vi "Current_Training_UI.vi"() -> ()   [LabVIEW 2021]
uses:
  SerialVIs/Processors.ctl
panel:
  out "Motor Value":i32
  in  "Quit":bool
  out "Training String":string
  out "Tab Control":enum32{"Welcome", "View", "Train"}(tab)
  in  "Ready":bool
  out "new picture":picture
  out "Motor Position View":dbl(knob) scale=0.0..180.0 scale format="%^#_3g"
  in  "TRAIN":bool
  out "Light Intensity % View":dbl(slide) scale=0.0..100.0
  out "?":u32(colorbox)
  out "new picture 4":picture
  in  "Done":bool
  in  "Motor Position":dbl(knob) scale=0.0..180.0 scale format="%^#_3g"
  out "Light Intensity %":dbl(slide) scale=0.0..100.0
  in  "Training Data":bool
  in  "Upload":bool
  out "Light Intensity 2":u32(colorbox)
  out "new picture 2":picture
  out "new picture 3":picture
  in  "Done 2":bool
  out "Upload String":string
  out "concatenated string":string
  out "read buffer":string
  out "Motor":string
  out "Sensor":string
  out "Type":string
  out "Name":string
  out "read terminal buffer - view":string
  out "Serial Settings:Number of Bytes at Serial Port 2":u32
  out "read buffer 2":string
  # "help button pops up a help message"
  # "1"
  # "2"
  # "5"
  # "3"
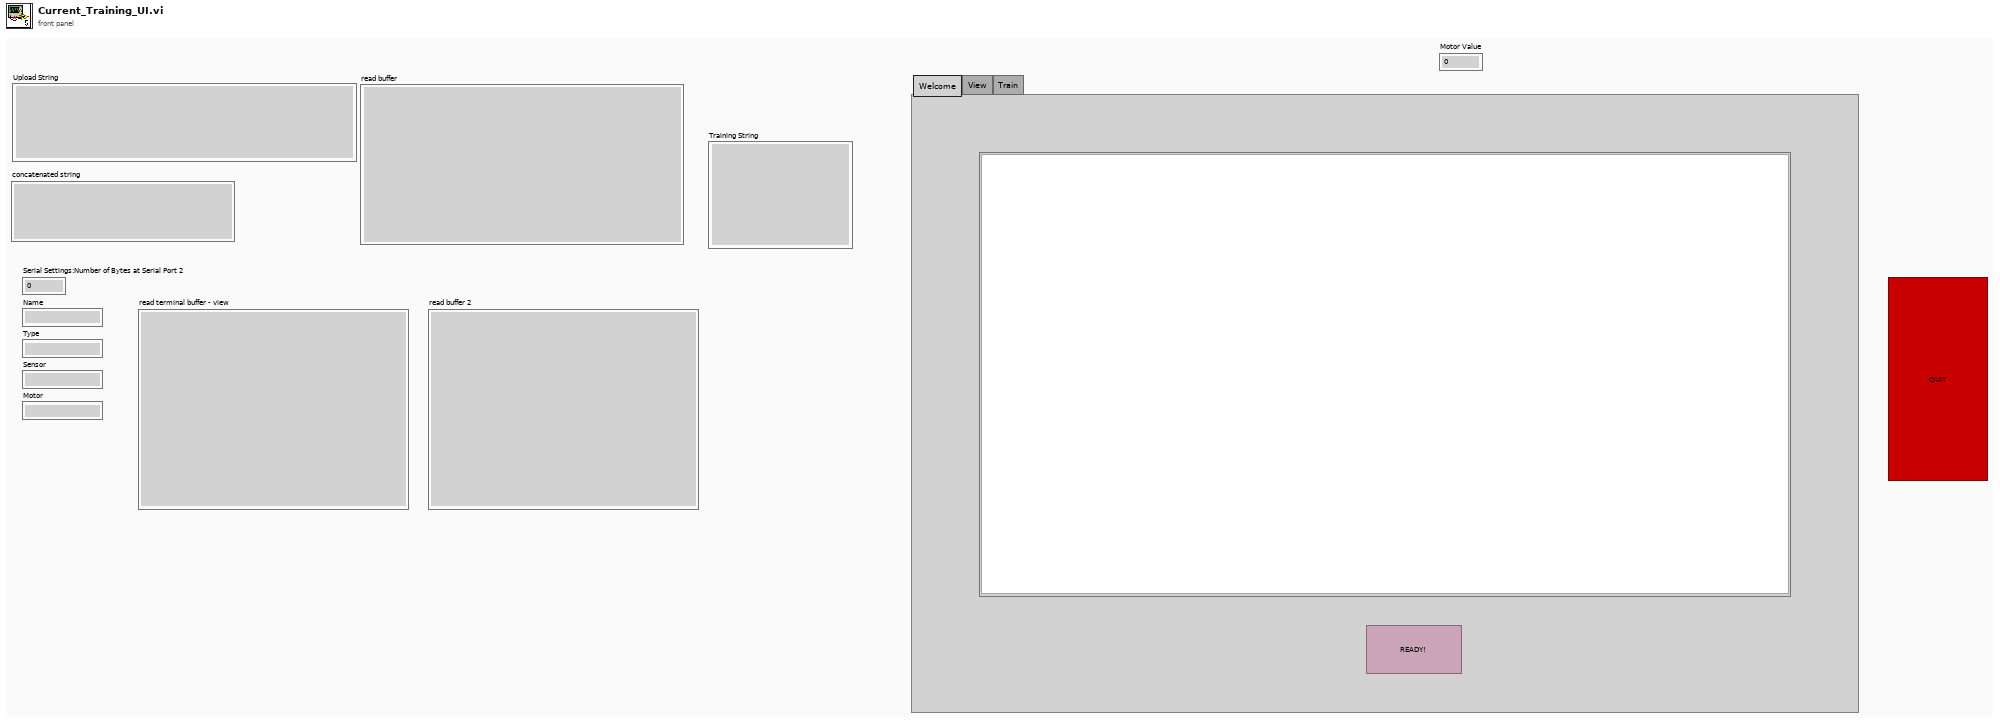
[diagram p1: front panel]
types:
  T1 = typedef "Processors.ctl" = enum16{"SPIKE", "Pi", "Pi_ssh", "OpenMV"}
  T2 = typedef "PythonCtrl.ctl" = cluster{"session":refnum<k35>, "PyPath":path, "Processor":enum16{"SPIKE", "Pi", "Pi_ssh"}}
  T3 = typedef "imagedata.ctl" = cluster{"image type":i32, "image depth":i32, "image":u8[], "mask":u8[], "colors":u32[], "Rectangle":cluster{"left":i16, "top":i16, "right":i16, "bottom":i16}}
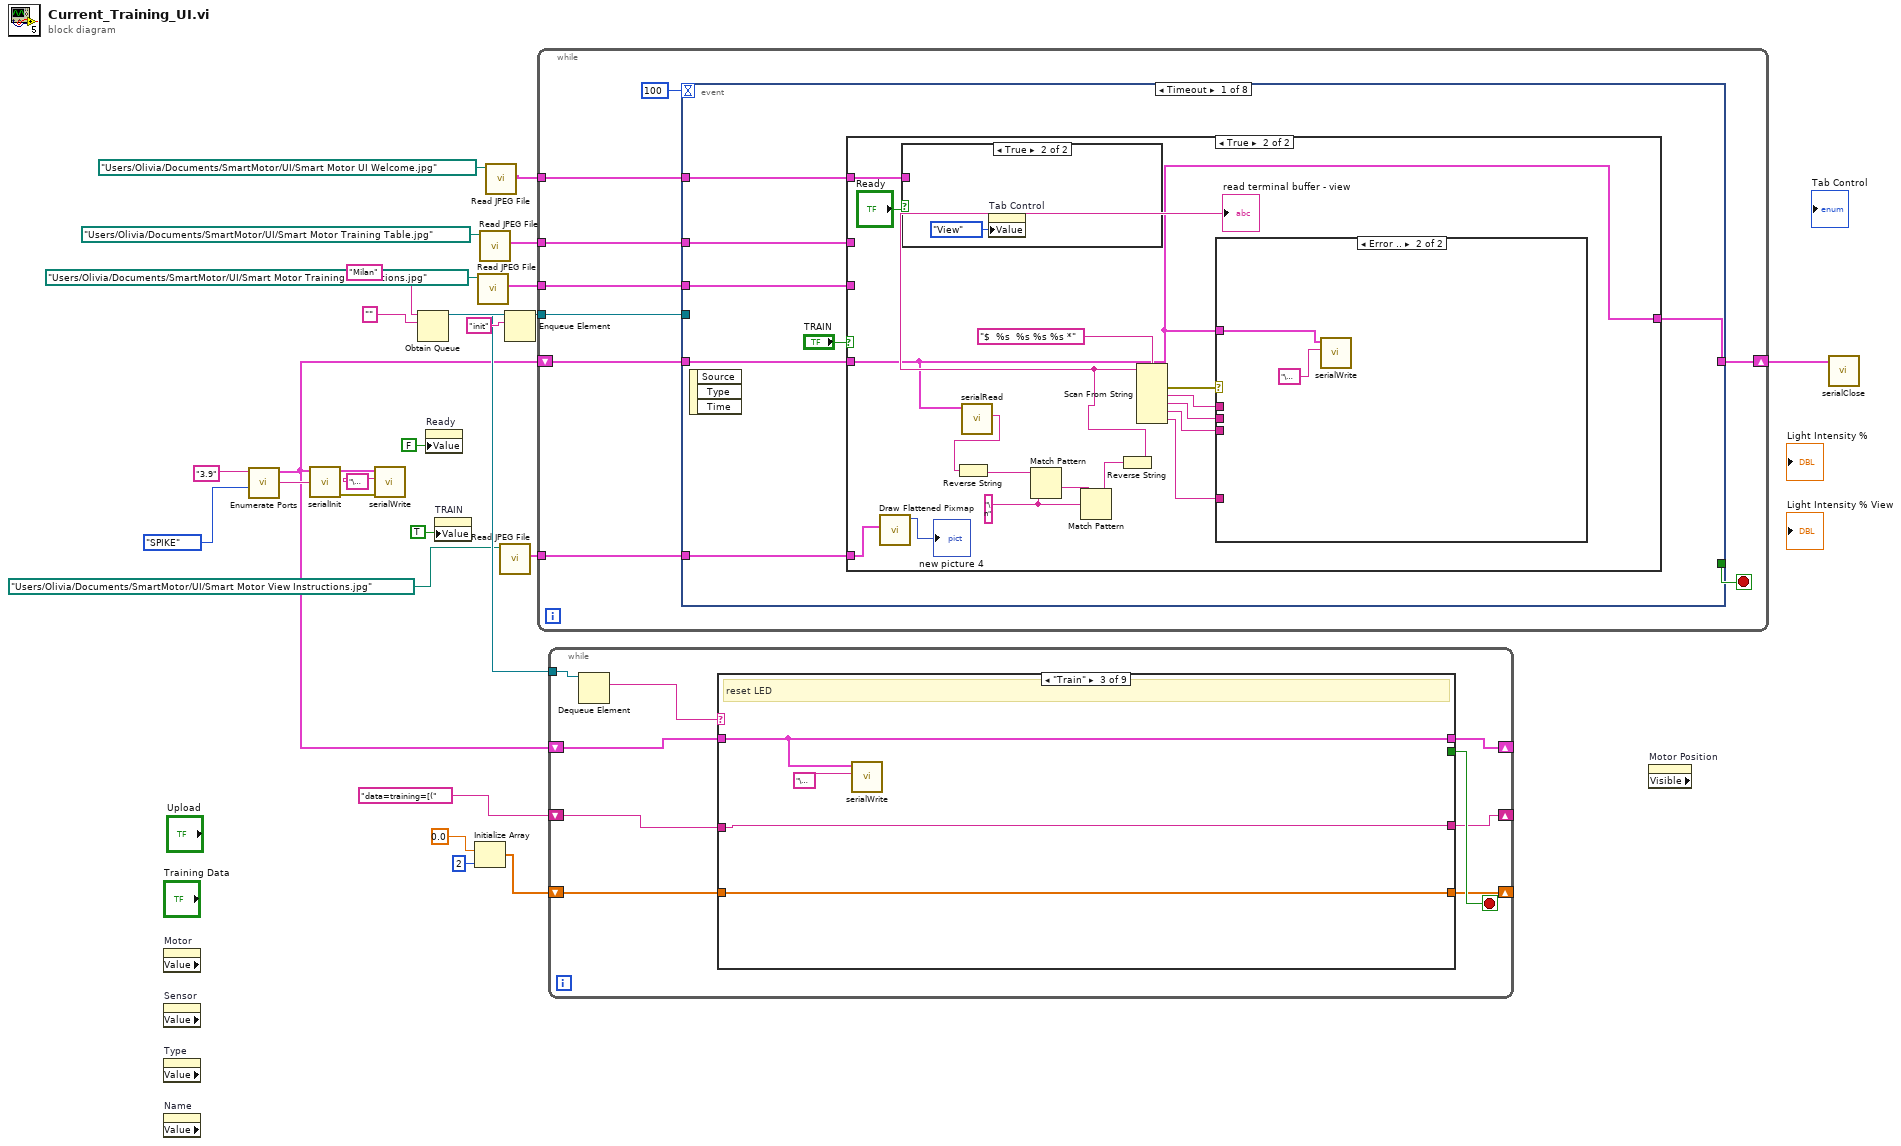
[diagram p0: block diagram]
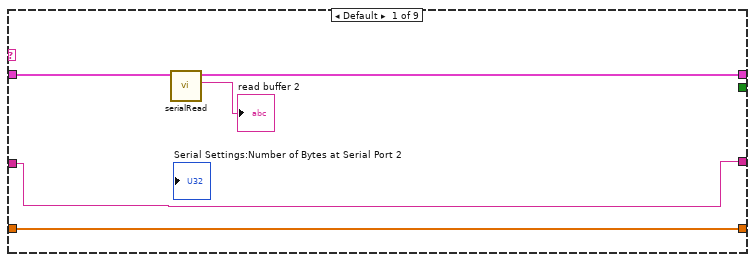
[diagram p2: hidden frame]
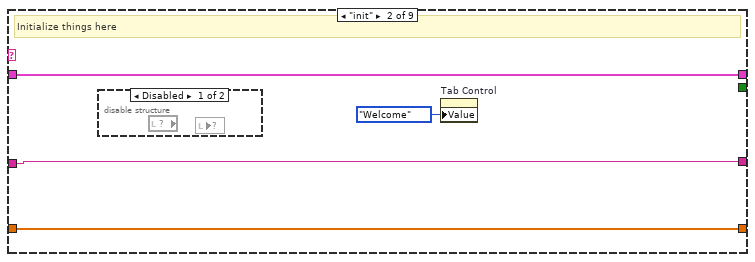
[diagram p3: hidden frame]
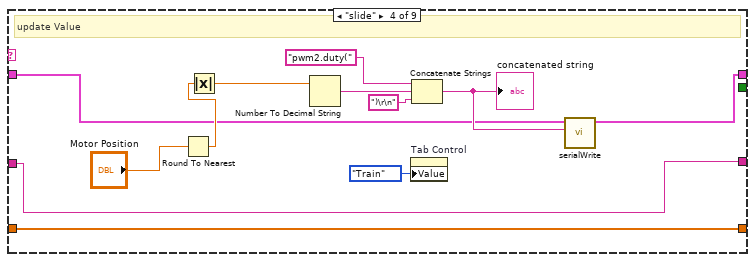
[diagram p5: hidden frame]
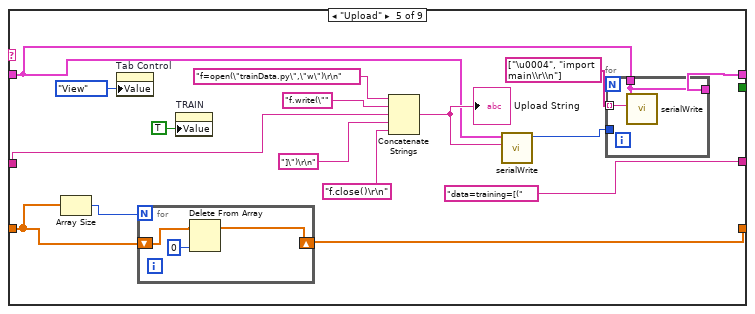
[diagram p6: hidden frame]
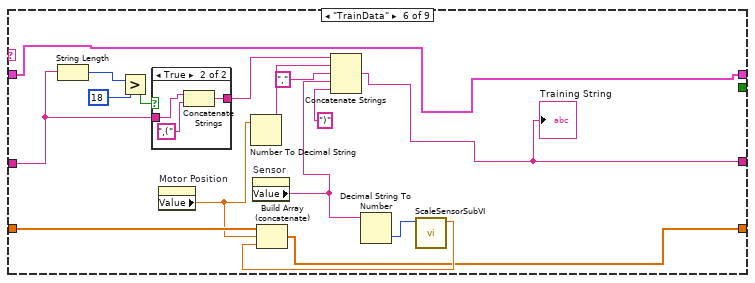
[diagram p7: hidden frame]
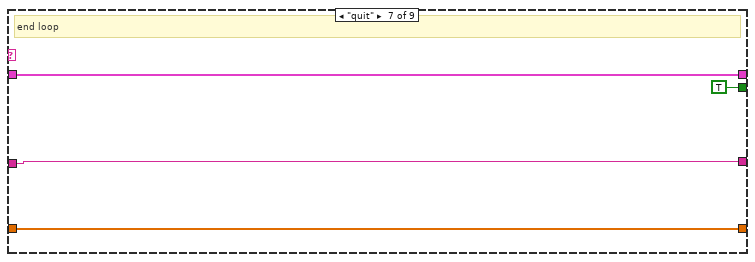
[diagram p9: hidden frame]
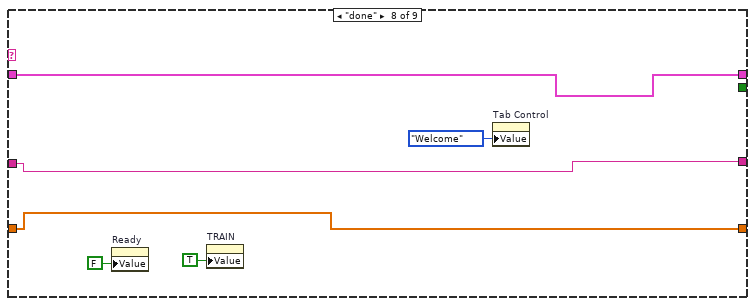
[diagram p10: hidden frame]
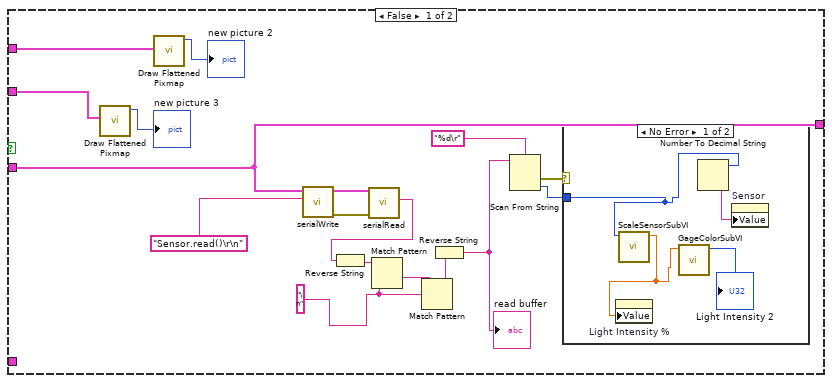
[diagram p12: hidden frame]
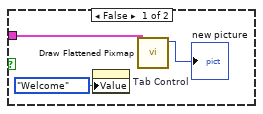
[diagram p14: hidden frame]
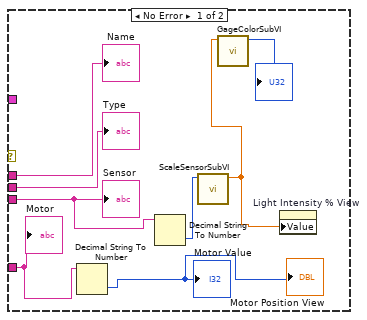
[diagram p15: hidden frame]
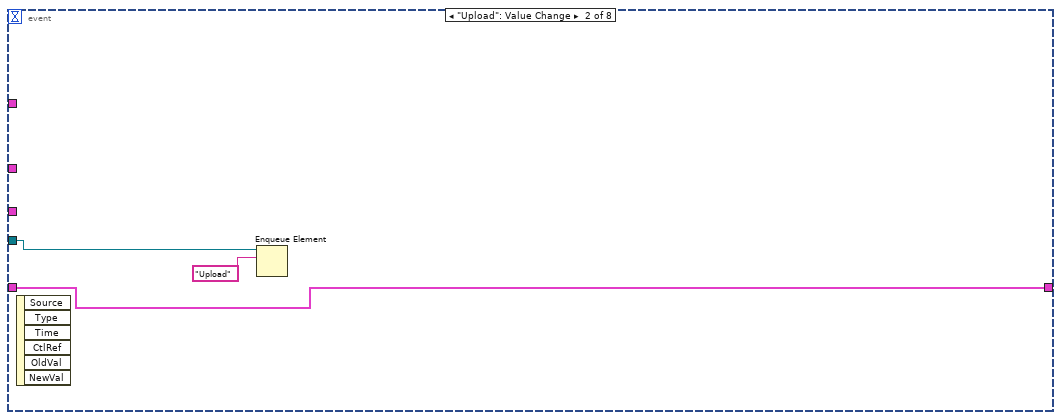
[diagram p16: hidden frame]
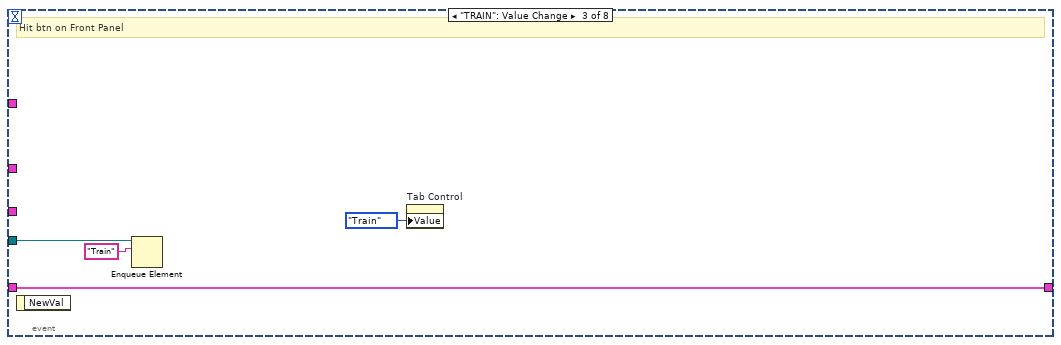
[diagram p17: hidden frame]
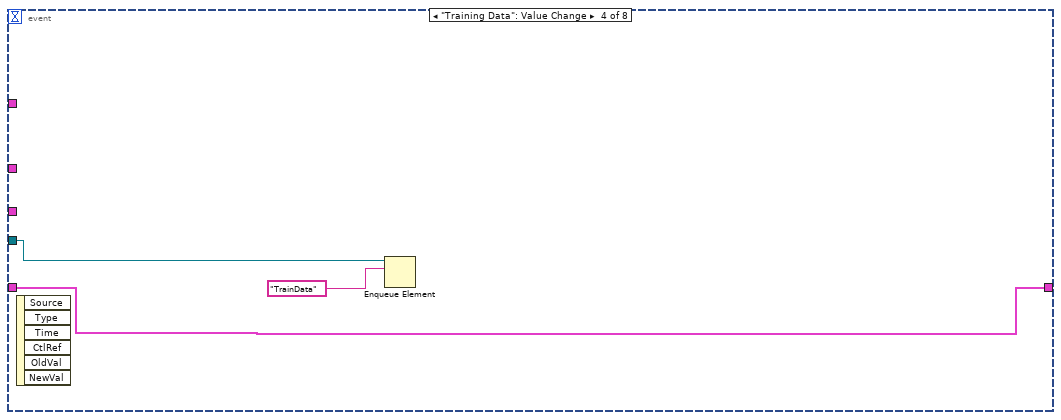
[diagram p18: hidden frame]
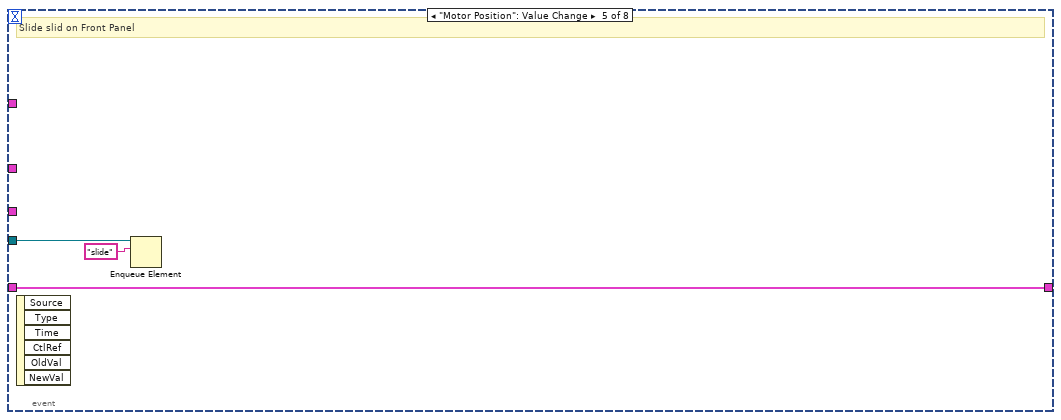
[diagram p19: hidden frame]
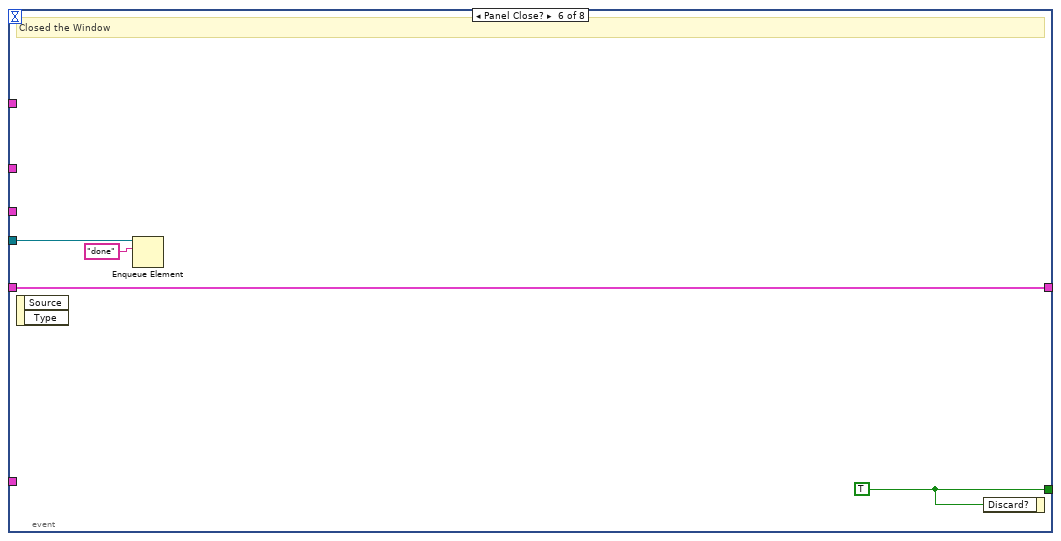
[diagram p20: hidden frame]
diagram:
  n1 = property on="Motor" class="Str" props=["Value"]() -> ()  [unwired: 2 in, 3 out]
  n2 = property on="Sensor" class="Str" props=["Value"]() -> ()  [unwired: 2 in, 3 out]
  n3 = property on="Type" class="Str" props=["Value"]() -> ()  [unwired: 2 in, 3 out]
  n4 = property on="Name" class="Str" props=["Value"]() -> ()  [unwired: 2 in, 3 out]
  n5 = call "Enumerate Ports.vi"("Processor"=Processors."SPIKE", "Python version"="3.9") -> ("guess"=w17:string, "Python"=w14:T2)  [unwired: 5 in, 3 out]
  n6 = call "serialInit.vi"("Port"=w17, "Python"=w14) -> ("error out"=w16:errorcluster)  [unwired: 8 in, 1 out]
  n7 = call "serialWrite.vi"("error in (no error)"=w16, "text"="\u0004" ("write buffer"), "Python"=w14) -> ()  [unwired: 7 in, 2 out]
  n8 = Obtain Queue(name (unnamed)="Milan", element data type="") -> (queue out=w26:refnum<queue>)  [unwired: 3 in, 2 out]
  n9 = property on="Ready" class="Bool (strict)"("Value"=FALSE ("Ready")) -> ()  [unwired: 2 in, 2 out]
  n10 = property on="TRAIN" class="Bool (strict)"("Value"=TRUE ("Train")) -> ()  [unwired: 2 in, 2 out]
  n11 = Initialize Array(0.0 ("element"), 2 ("dimension size")) -> (w2:dbl[])
  n12 = call <vilib>:"Read JPEG File.vi"("path to JPEG file"=path "/Users/Olivia/Documents/SmartMotor/UI/Smart Motor Training Instructions.jpg") -> ("image data"=w9:T3)  [unwired: 8 in, 2 out]
  n13 = call <vilib>:"Read JPEG File.vi"("path to JPEG file"=path "/Users/Olivia/Documents/SmartMotor/UI/Smart Motor Training Table.jpg") -> ("image data"=w11:T3)  [unwired: 8 in, 2 out]
  n14 = call <vilib>:"Read JPEG File.vi"("path to JPEG file"=path "/Users/Olivia/Documents/SmartMotor/UI/Smart Motor UI Welcome.jpg") -> ("image data"=w5:T3)  [unwired: 8 in, 2 out]
  n15 = call <vilib>:"Read JPEG File.vi"("path to JPEG file"=path "/Users/Olivia/Documents/SmartMotor/UI/Smart Motor View Instructions.jpg") -> ("image data"=w7:T3)  [unwired: 8 in, 2 out]
  n16 = Enqueue Element(queue=w26, element="init") -> (queue out=w22:refnum<queue>)  [unwired: 2 in, 2 out]
  n17 = while {
    tunnel: w22 -> [w35]
    shift-right: [w32] -> w13
    shift-left: w14 -> [w33]
    tunnel: w5 -> [w30]
    tunnel: w11 -> [w29]
    tunnel: w9 -> [w28]
    tunnel: w7 -> [w27]
    stop <- w34 stop-if-true
    n18 = event shown="[0] Timeout" {
      selector: _ -> [_ _ _ _ _ _ _ _]
      dyn-events: _ -> [_ _ _ _ _ _ _ _]
      timeout: 100 -> [_ _ _ _ _ _ _ _]
      tunnel: w35 -> [_ w96 w99 w102 w105 w109 w113 w116]
      tunnel: [_ _ _ _ _ w108 TRUE ("Discard?") _] -> w34
      tunnel: w33 -> [w40 w94 w98 w101 w104 w107 w111 w115]
      tunnel: [w41 w94 w98 w101 w104 w107 w111 w115] -> w32
      tunnel: w30 -> [w39 _ _ _ _ _ _ _]
      tunnel: w29 -> [w38 _ _ _ _ _ _ _]
      tunnel: w28 -> [w37 _ _ _ _ _ _ _]
      tunnel: w27 -> [w36 _ _ _ _ _ _ _]
      event Timeout {
        n19 = event-data() -> ()  [unwired: 1 in, 3 out]
        n20 = case shown="True" "TRAIN" {
          tunnel: w40 -> [w53 w63]
          tunnel: [w53 w63] -> w41
          tunnel: w39 -> [_ w66]
          tunnel: w38 -> [w45 _]
          tunnel: w37 -> [w43 _]
          tunnel: w36 -> [_ w64]
          frame False {
            w50 = "\n" ("regular expression")
            n21 = call <vilib>:"Draw Flattened Pixmap.vi"("image data"=w43) -> ("new picture"=→"new picture 3":picture)  [unwired: 8 in]
            n22 = call <vilib>:"Draw Flattened Pixmap.vi"("image data"=w45) -> ("new picture"=→"new picture 2":picture)  [unwired: 8 in]
            n23 = call "serialWrite.vi"("text"="Sensor.read()\r\n" ("write buffer"), "Python"=w53) -> ("error out"=w54:errorcluster)  [unwired: 8 in, 1 out]
            n24 = call "serialRead.vi"("error in (no error)"=w54, "Python"=w53) -> ("Reply"=w47:string)  [unwired: 7 in, 2 out]
            n25 = Reverse String(1:w47) -> (0:w52:string)
            n26 = Match Pattern(string=w52, regular expression=w50) -> (after substring=w51:string)  [unwired: 1 in, 3 out]
            n27 = Match Pattern(string=w51, regular expression=w50) -> (before substring=w49:string)  [unwired: 1 in, 3 out]
            n28 = Reverse String(1:w49) -> (0:w48:string)
            "read buffer" <- w48
            n29 = Scan From String(format string="%d\r", input string=w48) -> (error out=w58:errorcluster, output 1=w57:i32)  [unwired: 3 in, 2 out]
            n30 = case shown="No Error" w58 {
              tunnel: w57 -> [w60 _]
              frame No Error {
                n31 = call "ScaleSensorSubVI.vi"("Numeric in"=w60) -> ("Numeric out"=w59:dbl)  [unwired: 10 in]
                n32 = property on="Light Intensity %" class="Slide (strict)"("Value"=w59) -> ()  [unwired: 2 in, 2 out]
                n33 = call "GageColorSubVI.vi"("Numeric"=w59) -> ("Color Box"=→"Light Intensity 2":u32)  [unwired: 10 in]
                n34 = Number To Decimal String(number=w60) -> (decimal integer string=w62:string)  [unwired: 1 in]
                n35 = property on="Sensor" class="Str"("Value"=w62) -> ()  [unwired: 2 in, 2 out]
              }
              frame Error {
              }
            }
          }
          frame True {
            w70 = "\n" ("regular expression")
            n36 = call <vilib>:"Draw Flattened Pixmap.vi"("image data"=w64) -> ("new picture"=→"new picture 4":picture)  [unwired: 8 in]
            n37 = case shown="True" "Ready" {
              tunnel: w66 -> [w81 _]
              frame False {
                n38 = property on="Tab Control" class="TabCtl (strict)"("Value"=enum32{"Welcome", "View", "Train"}."Welcome" ("Tab Control")) -> ()  [unwired: 2 in, 2 out]
                n39 = call <vilib>:"Draw Flattened Pixmap.vi"("image data"=w81) -> ("new picture"=→"new picture":picture)  [unwired: 8 in]
              }
              frame True {
                n40 = property on="Tab Control" class="TabCtl (strict)"("Value"=enum32{"Welcome", "View", "Train"}."View" ("Tab Control")) -> ()  [unwired: 2 in, 2 out]
              }
            }
            n41 = call "serialRead.vi"("Python"=w63) -> ("Reply"=w73:string)  [unwired: 8 in, 2 out]
            n42 = Reverse String(1:w73) -> (0:w72:string)
            n43 = Match Pattern(string=w72, regular expression=w70) -> (after substring=w71:string)  [unwired: 1 in, 3 out]
            n44 = Match Pattern(string=w71, regular expression=w70) -> (before substring=w69:string)  [unwired: 1 in, 3 out]
            n45 = Reverse String(1:w69) -> (0:w68:string)
            "read terminal buffer - view" <- w68
            n46 = Scan From String(format string="$  %s  %s %s %s *", input string=w68) -> (error out=w79:errorcluster, output 1=w75:string, output 2=w76:string, output 3=w77:string, output 4=w78:string)  [unwired: 6 in, 2 out]
            n47 = case shown="Error .." w79 {
              tunnel: w75 -> [w91 _]
              tunnel: w76 -> [w90 _]
              tunnel: w77 -> [w89 _]
              tunnel: w78 -> [w85 _]
              tunnel: w63 -> [_ w93]
              frame No Error {
                n48 = Decimal String To Number(string=w85) -> (number=→"Motor Value" →"Motor Position View":i32)  [unwired: 2 in, 1 out]
                n49 = Decimal String To Number(string=w89) -> (number=w88:i32)  [unwired: 2 in, 1 out]
                n50 = call "ScaleSensorSubVI.vi"("Numeric in"=w88) -> ("Numeric out"=w86:dbl)  [unwired: 10 in]
                n51 = call "GageColorSubVI.vi"("Numeric"=w86) -> ("Color Box"=→"?":u32)  [unwired: 10 in]
                n52 = property on="Light Intensity % View" class="Slide (strict)"("Value"=w86) -> ()  [unwired: 2 in, 2 out]
                "Name" <- w91
                "Type" <- w90
                "Sensor" <- w89
                "Motor" <- w85
              }
              frame Error {
                n53 = call "serialWrite.vi"("text"="\u0003", "Python"=w93) -> ()  [unwired: 8 in, 2 out]
              }
            }
          }
        }
      }
      event "Upload": Value Change {
        n54 = event-data() -> ()  [unwired: 1 in, 6 out]
        n55 = Enqueue Element(queue=w96, element="Upload") -> ()  [unwired: 2 in, 3 out]
      }
      event "TRAIN": Value Change {
        # "Hit btn on Front Panel"
        n56 = event-data() -> ()  [unwired: 1 in, 1 out]
        n57 = Enqueue Element(queue=w99, element="Train") -> ()  [unwired: 2 in, 3 out]
        n58 = property on="Tab Control" class="TabCtl (strict)"("Value"=enum32{"Welcome", "View", "Train"}."Train" ("Tab Control")) -> ()  [unwired: 2 in, 2 out]
      }
      event "Training Data": Value Change {
        n59 = event-data() -> ()  [unwired: 1 in, 6 out]
        n60 = Enqueue Element(queue=w102, element="TrainData") -> ()  [unwired: 2 in, 3 out]
      }
      event "Motor Position": Value Change {
        # "Slide slid on Front Panel"
        n61 = event-data() -> ()  [unwired: 1 in, 6 out]
        n62 = Enqueue Element(queue=w105, element="slide") -> ()  [unwired: 2 in, 3 out]
      }
      event Panel Close? {
        w108 = TRUE ("Discard?")
        # "Closed the Window"
        n63 = event-data() -> ()  [unwired: 1 in, 2 out]
        n64 = Enqueue Element(queue=w109, element="done") -> ()  [unwired: 2 in, 3 out]
        n65 = event-data("Discard?"=w108) -> ()  [unwired: 1 in, 1 out]
      }
      event "Quit": Value Change {
        # "hit Done btn"
        n66 = event-data() -> ()  [unwired: 1 in, 2 out]
        n67 = Enqueue Element(queue=w113, element="quit") -> ()  [unwired: 2 in, 3 out]
      }
      event "Done": Value Change {
        n68 = event-data() -> ()  [unwired: 1 in, 6 out]
        n69 = Enqueue Element(queue=w116, element="done") -> ()  [unwired: 2 in, 3 out]
      }
    }
  }
  n70 = while {
    tunnel: w22 -> [w126]
    shift-right: [w122] -> _
    shift-left: w14 -> [w123]
    shift-right: [w120] -> _
    shift-left: "data=training=[(" -> [w121]
    shift-right: [w118] -> _
    shift-left: w2 -> [w119]
    stop <- w124 stop-if-true
    n71 = Dequeue Element(queue=w126) -> (element=w125:string)  [unwired: 2 in, 3 out]
    n72 = case shown="\"Train\"" w125 {
      tunnel: [_ _ _ _ _ _ TRUE ("Discard?") _ _] -> w124
      tunnel: w123 -> [w128 w134 w137 w141 w157 w183 w193 w197 w203]
      tunnel: [w128 w134 w137 w141 w155 w183 w193 w197 w203] -> w122
      tunnel: w121 -> [w130 w133 w138 w143 w163 w178 w192 w200 w202]
      tunnel: [w130 w133 w138 w143 "data=training=[(" w177 w192 w200 w202] -> w120
      tunnel: w119 -> [w127 w132 w135 w139 w150 w176 w191 w198 w201]
      tunnel: [w127 w132 w135 w139 w151 w171 w191 w198 w201] -> w118
      frame Default {
        n73 = call "serialRead.vi"("Python"=w128) -> ("Reply"=→"read buffer 2":string)  [unwired: 8 in, 2 out]
      }
      frame "init" {
        # "Initialize things here"
        n74 = disable-structure shown="Disabled" {
          frame Disabled {
            n75 = local read item#-1() -> ()  [unwired: 1 out]
            n76 = local read item#-1() -> ()  [unwired: 1 in]
          }
          frame Enabled {
          }
        }
        n77 = property on="Tab Control" class="TabCtl (strict)"("Value"=enum32{"Welcome", "View", "Train"}."Welcome" ("Tab Control")) -> ()  [unwired: 2 in, 2 out]
      }
      frame "Train" {
        # "reset LED"
        n78 = call "serialWrite.vi"("text"="\u0003" ("write buffer"), "Python"=w137) -> ()  [unwired: 8 in, 2 out]
      }
      frame "slide" {
        # "update Value"
        n79 = Round To Nearest(number="Motor Position") -> (nearest integer value=w144:dbl)
        n80 = Absolute Value(x=w144) -> (abs(x)=w146:dbl)
        n81 = Number To Decimal String(number=w146) -> (decimal integer string=w148:string)  [unwired: 1 in]
        n82 = property on="Tab Control" class="TabCtl (strict)"("Value"=enum32{"Welcome", "View", "Train"}."Train" ("Tab Control")) -> ()  [unwired: 2 in, 2 out]
        n83 = Concatenate Strings("pwm2.duty(", w148, ")\r\n" ("string")) -> (w142:string)
        "concatenated string" <- w142
        n84 = call "serialWrite.vi"("text"=w142, "Python"=w141) -> ()  [unwired: 8 in, 2 out]
      }
      frame "Upload" {
        n85 = Array Size(array=w150) -> (size(s)=w152:i32)
        n86 = property on="Tab Control" class="TabCtl (strict)"("Value"=enum32{"Welcome", "View", "Train"}."View" ("Tab Control")) -> ()  [unwired: 2 in, 2 out]
        n87 = for {
          N: w152 -> [_]
          shift-right: [w167] -> w151
          shift-left: w150 -> [w166]
          n88 = Delete From Array(array=w166, index=0) -> (array with subset deleted=w167:dbl[])  [unwired: 1 in, 1 out]
        }
        n89 = property on="TRAIN" class="Bool (strict)"("Value"=TRUE ("TRAIN")) -> ()  [unwired: 2 in, 2 out]
        n90 = Concatenate Strings("f=open(\"trainData.py\",\"w\")\r\n" ("string"), "f.write(\"" ("string"), w163, "]\")\r\n" ("string"), "f.close()\r\n" ("string")) -> (w159:string)
        "Upload String" <- w159
        n91 = call "serialWrite.vi"("text"=w159, "Python"=w157) -> ("Num loops"=w153:i32)  [unwired: 8 in, 1 out]
        n92 = for {
          tunnel: w157 -> [w169]
          tunnel: string[] ["\u0004", "import main\\r\\n"] -> [w170] mode=indexing
          tunnel: [w169] -> w155
          tunnel: w153 -> [_]
          n93 = call "serialWrite.vi"("text"=w170, "Python"=w169) -> ()  [unwired: 8 in, 2 out]
        }
      }
      frame "TrainData" {
        n94 = String Length(string=w178) -> (length=w182:i32)
        n95 = Greater?(x=w182, y=18) -> (0:w180:bool)
        n96 = case shown="True" w180 {
          tunnel: w178 -> [w187 w189]
          tunnel: [w187 w188] -> w179
          frame False {
          }
          frame True {
            n97 = Concatenate Strings(w189, ",(" ("string")) -> (w188:string)
          }
        }
        n98 = property on="Motor Position" class="Knob (strict)"() -> ("Value"=w175:dbl)  [unwired: 2 in, 2 out]
        n99 = Number To Decimal String(number=w175) -> (decimal integer string=w186:string)  [unwired: 1 in]
        n100 = property on="Sensor" class="Str"() -> ("Value"=w174:string)  [unwired: 2 in, 2 out]
        n101 = Concatenate Strings(w179, w186, "," ("string"), w174, ")" ("string")) -> (w177:string)
        "Training String" <- w177
        n102 = Decimal String To Number(string=w174) -> (number=w173:i32)  [unwired: 2 in, 1 out]
        n103 = call "ScaleSensorSubVI.vi"("Numeric in"=w173) -> ("Numeric out"=w172:dbl)  [unwired: 10 in]
        n104 = Build Array (concatenate)(w176, w175, w172) -> (w171:dbl[])
      }
      frame "quit" {
        # "end loop"
      }
      frame "done" {
        n105 = property on="Ready" class="Bool (strict)"("Value"=FALSE ("Ready")) -> ()  [unwired: 2 in, 2 out]
        n106 = property on="TRAIN" class="Bool (strict)"("Value"=TRUE ("TRAIN")) -> ()  [unwired: 2 in, 2 out]
        n107 = property on="Tab Control" class="TabCtl (strict)"("Value"=enum32{"Welcome", "View", "Train"}."Welcome" ("Tab Control")) -> ()  [unwired: 2 in, 2 out]
      }
      frame "" {
      }
    }
  }
  n108 = property on="Motor Position" class="Knob (strict)" props=["Visible"]() -> ()  [unwired: 2 in, 3 out]
  n109 = call "serialClose.vi"("Python in"=w13) -> ()  [unwired: 10 in, 1 out]
